vi "acc_gyro_motor_logger.vi"() -> ()   [LabVIEW 2012]
uses:
  <vilib>/Instr/_visa.llb/VISA Configure Serial Port (Instr).vi
  acc_gyro_data.ctl
panel:
  out "return count":u32
  in  "stop 2":bool
  out "Encoder":u8[](graph)
  in  "amp":dbl
  in  "freq":dbl
  in  "Send":bool
  in  "encoder counts per rev":dbl=2048.0
  in  "Motor serial port":refnum<visa-resource-name>="COM3"
  out "Rate":dbl[unit]
  out "Accelerometer":waveform(dbl)[](graph)
  out "Gyro":waveform(dbl)[](graph)
  in  "accel range (m/s2)":dbl(ring)=8.0 items=["2"=2.0, "4"=4.0, "8"=8.0, "16"=16.0]
  in  "gyro range (deg/s)":dbl(ring)=250.0 items=["250"=250.0, "500"=500.0, "1000"=1000.0, "2000"=2000.0]
  in  "Accelometer serial port":refnum<visa-resource-name>="COM3"
  in  "stop":bool
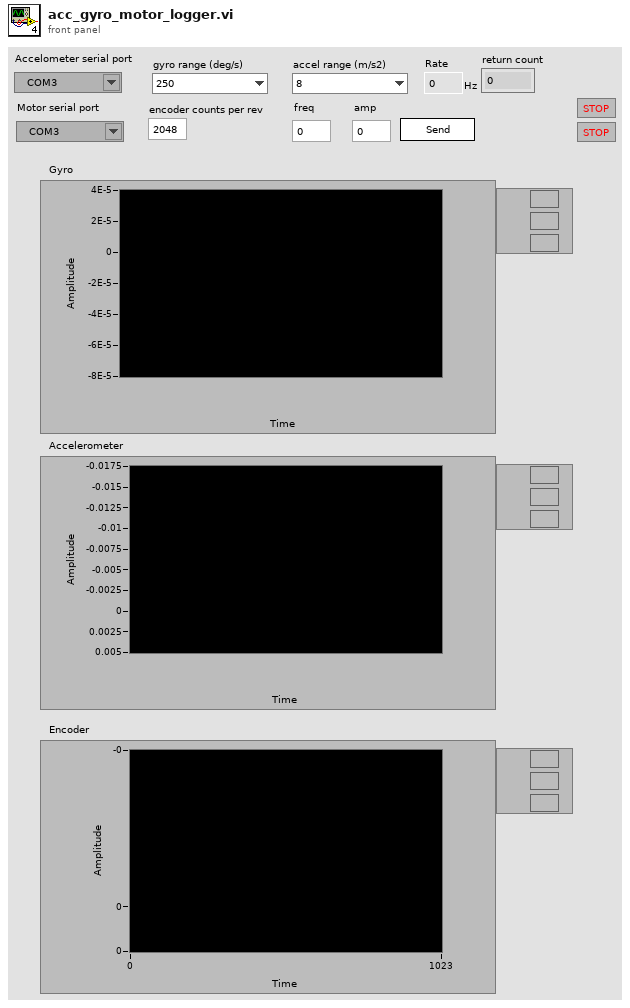
[diagram p1: front panel]
types:
  T1 = typedef "acc_gyro_data.ctl" = cluster{"milliseconds":u64, "gyro_x":dbl, "gyro_y":dbl, "gyro_z":dbl, "acc_x":dbl, "acc_y":dbl, "acc_z":dbl}
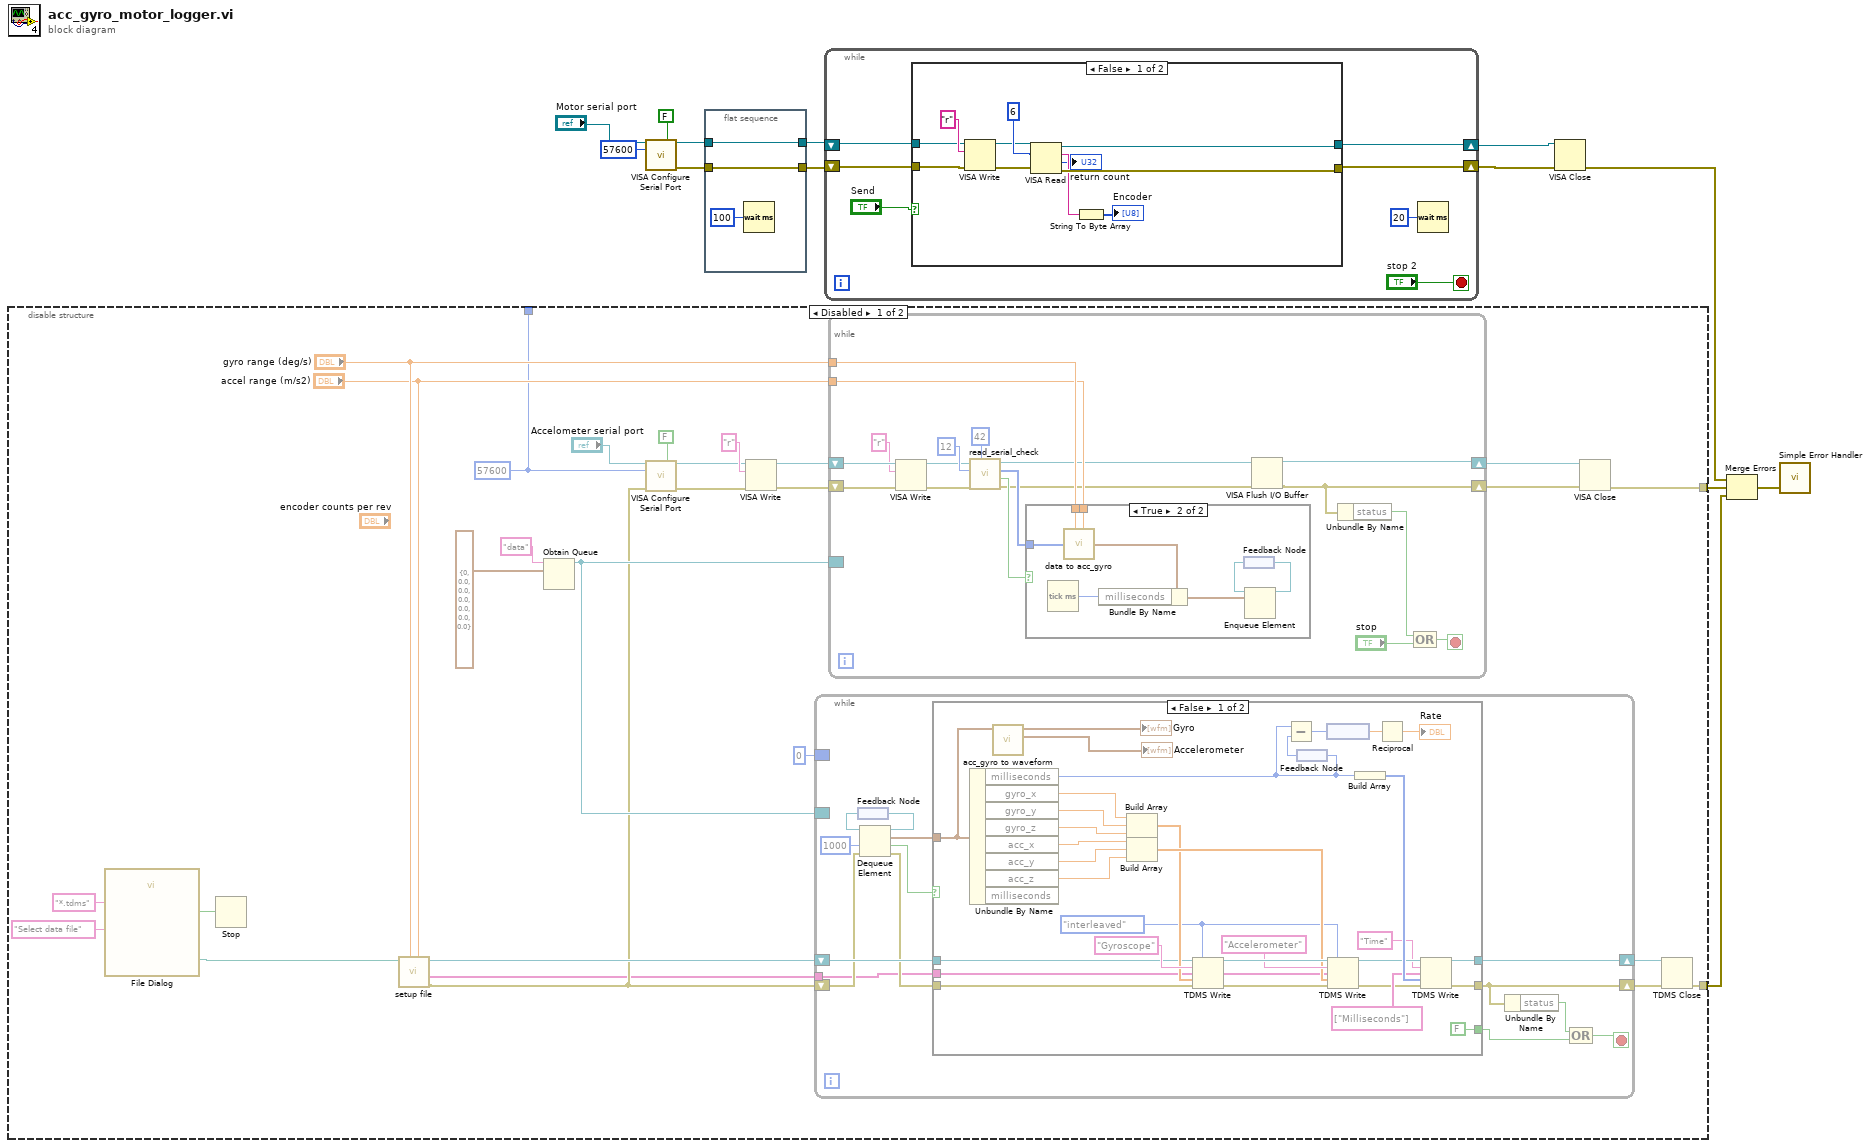
[diagram p0: block diagram]
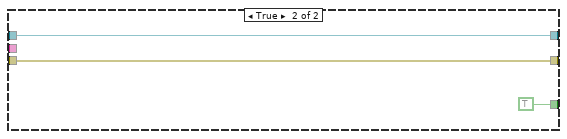
[diagram p2: hidden frame]
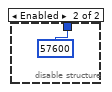
[diagram p4: hidden frame]
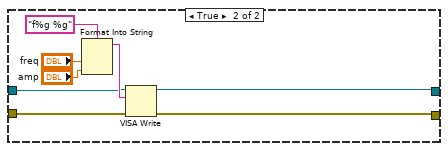
[diagram p5: hidden frame]
diagram:
  n1 = disable-structure shown="Disabled" {
    disable-tunnel: [w27 _] -> w13
    disable-tunnel: [w26 _] -> w12
    disable-tunnel: [w14 u32 57600 ("Baud rate")] -> _
    frame Disabled {
      w14 = u32 57600 ("Baud rate")
      n2 = call "File Dialog"("prompt"="Select data file", "pattern (all files)"="*.tdms") -> ("selected path"=w34:path, "cancelled"=w33:bool)  [unwired: 10 in, 2 out]
      n3 = Stop(stop? (T)=w33) -> ()
      n4 = call "setup file.vi"("accel range"="accel range (m/s2)", "gyro range"="gyro range (deg/s)", "selected path"=w34) -> ("error out"=w24:errorcluster, "channel names"=w21:string[], "tdms file out"=w25:refnum<k34>)  [unwired: 6 in]
      n5 = Obtain Queue(name (unnamed)="data", element data type=T1 {"milliseconds"=0, "gyro_x"=0.0, "gyro_y"=0.0, "gyro_z"=0.0, "acc_x"=0.0, "acc_y"=0.0, "acc_z"=0.0} ("acc gyro data")) -> (queue out=w32:refnum<queue>)  [unwired: 3 in, 2 out]
      n6 = call-poly "VISA Configure Serial Port"("VISA resource name"="Accelometer serial port", "Enable Termination\nChar (T)"=FALSE ("Enable Termination\nChar (T)"), "baud rate (9600)"=w14, "error in (no error)"=w24) -> ("VISA resource name out"=w18:refnum<visa-resource-name>, "error out"=w17:errorcluster)  [unwired: 10 in]
      n7 = VISA Write(VISA resource name=w18, write buffer="r", error in (no error)=w17) -> (VISA resource name out=w16:refnum<visa-resource-name>, error out=w15:errorcluster)  [unwired: 1 out]
      n8 = while {
        border: w32 -> [_]
        shift-right: [w45] -> w29
        shift-left: w24 -> [w48]
        shift-right: [w50] -> w28
        shift-left: w25 -> [w51]
        tunnel: w21 -> [w41]
        border: u64 0 ("milliseconds") -> [_]
        stop <- w42 stop-if-true
        n9 = feedback #1() -> (w54:refnum<queue>)
        n10 = Dequeue Element(queue=w54, timeout in ms (-1)=1000, error in (no error)=w48) -> (queue out=w53:refnum<queue>, element=w52:T1, timed out?=w46:bool, error out=w47:errorcluster)
        n11 = feedback-in #1(w53) -> ()
        n12 = case shown="False" w46 {
          tunnel: w52 -> [w72 _]
          tunnel: [w63 w88] -> w45
          tunnel: w51 -> [w61 w89]
          tunnel: [w62 w89] -> w50
          tunnel: w47 -> [w64 w88]
          tunnel: [FALSE TRUE] -> w43
          tunnel: w41 -> [w69 _]
          frame False {
            w60 = enum16{"decimated", "interleaved"}."interleaved" ("data layout (0:decimated)")
            n13 = Unbundle By Name(w72) -> ("milliseconds"=w59:u64, "gyro_x"=w87:dbl, "gyro_y"=w86:dbl, "gyro_z"=w85:dbl, "acc_x"=w84:dbl, "acc_y"=w83:dbl, "acc_z"=w82:dbl)  [unwired: 1 out]
            n14 = call "acc_gyro to waveform.vi"("acc gyro data"=w72) -> ("accel plot"=→"Accelerometer":waveform(dbl)[], "gyro plot"=→"Gyro":waveform(dbl)[])  [unwired: 9 in]
            n15 = Build Array(w87, w86, w85) -> (w73:dbl[])
            n16 = Build Array(w84, w83, w82) -> (w77:dbl[])
            n17 = TDMS Write(0:w61, 1:w60, 5:"Gyroscope" ("group name (Untitled)"), 7:w69, 9:w73, 11:w64) -> (4:w80:refnum<k34>, 8:w68:string[], 15:w79:errorcluster)  [unwired: 1 out]
            n18 = feedback #2() -> (w58:u64)
            n19 = Subtract(x=w59, y=w58) -> (x-y=w57:u64)
            n20 = feedback-in #2(w59) -> ()
            n21 = node(w57) -> (w56:dbl[unit])
            n22 = TDMS Write(0:w80, 1:w60, 5:"Accelerometer" ("group name (Untitled)"), 7:w68, 9:w77, 11:w79) -> (4:w67:refnum<k34>, 15:w66:errorcluster)  [unwired: 2 out]
            n23 = Build Array(w59) -> (w76:u64[])
            n24 = Reciprocal(x=w56) -> (1/x=→"Rate":dbl[unit])
            n25 = TDMS Write(0:w67, 5:"Time" ("group name (Untitled)"), 7:string[] ["Milliseconds"] ("channel name(s) in (Untitled)"), 9:w76, 11:w66) -> (4:w62:refnum<k34>, 15:w63:errorcluster)  [unwired: 1 in, 2 out]
          }
          frame True {
          }
        }
        n26 = Unbundle By Name(w45) -> ("status"=w44:bool)
        n27 = Compound Arithmetic op=OR(w44, w43) -> (w42:bool)
      }
      n28 = while {
        tunnel: "gyro range (deg/s)" -> [w103]
        tunnel: "accel range (m/s2)" -> [w102]
        border: w32 -> [_]
        shift-right: [w91] -> w31
        shift-left: w15 -> [w99]
        shift-right: [w93] -> w30
        shift-left: w16 -> [w108]
        stop <- w96 stop-if-true
        n29 = VISA Write(VISA resource name=w108, write buffer="r", error in (no error)=w99) -> (VISA resource name out=w101:refnum<visa-resource-name>, error out=w98:errorcluster)  [unwired: 1 out]
        n30 = call "read_serial_check.vi"("checkval"=u8 42, "error in (no error)"=w98, "byte count"=u32 12, "VISA resource name"=w101) -> ("error out"=w92:errorcluster, "good"=w105:bool, "data"=w104:u8[], "VISA resource out"=w94:refnum<visa-resource-name>)  [unwired: 4 in]
        n31 = case shown="True" w105 {
          tunnel: w104 -> [_ w116]
          tunnel: w103 -> [_ w115]
          tunnel: w102 -> [_ w114]
          frame False {
          }
          frame True {
            n32 = Tick Count (ms)() -> (millisecond timer value=w111:u32)
            n33 = call "data to acc_gyro.vi"("byte array"=w116, "gyro range (deg/s)"=w115, "accel range (m/s2)"=w114) -> ("acc gyro data"=w110:T1)
            n34 = Bundle By Name(cluster=w110, "milliseconds"=w111) -> (w109:T1)
            n35 = feedback #3() -> (w112:refnum<queue>)
            n36 = Enqueue Element(queue=w112, element=w109) -> (queue out=w113:refnum<queue>)  [unwired: 2 in, 2 out]
            n37 = feedback-in #3(w113) -> ()
          }
        }
        n38 = VISA Flush I/O Buffer(VISA resource name=w94, error in (no error)=w92) -> (VISA resource name out=w93:refnum<visa-resource-name>, error out=w91:errorcluster)  [unwired: 1 in]
        n39 = Unbundle By Name(w91) -> ("status"=w95:bool)
        n40 = Compound Arithmetic op=OR(w95, "stop") -> (w96:bool)
      }
      n41 = VISA Close(VISA resource name=w30, error in (no error)=w31) -> (error out=w27:errorcluster)
      n42 = TDMS Close(8:w29, 11:w28) -> (0:w26:errorcluster)  [unwired: 1 out]
    }
    frame Enabled {
    }
  }
  n43 = call-poly "VISA Configure Serial Port"("VISA resource name"="Motor serial port", "Enable Termination\nChar (T)"=FALSE ("Enable Termination\nChar (T)"), "baud rate (9600)"=u32 57600) -> ("VISA resource name out"=w5:refnum<visa-resource-name>, "error out"=w3:errorcluster)  [unwired: 11 in]
  n44 = flat-sequence {
    tunnel: w5 -> [w119]
    tunnel: [w119] -> w4
    tunnel: w3 -> [w118]
    tunnel: [w118] -> w2
    frame #0 {
      n45 = Wait (ms)(milliseconds to wait=u32 100) -> ()  [unwired: 1 out]
    }
  }
  n46 = while {
    shift-right: [w123] -> w7
    shift-left: w2 -> [w125]
    shift-right: [w124] -> w8
    shift-left: w4 -> [w126]
    stop <- "stop 2" stop-if-true
    n47 = case shown="False" "Send" {
      tunnel: w126 -> [w137 w142]
      tunnel: w125 -> [w136 w141]
      tunnel: [w132 w140] -> w124
      tunnel: [w131 w139] -> w123
      frame False {
        n48 = VISA Write(VISA resource name=w137, write buffer="r", error in (no error)=w136) -> (VISA resource name out=w134:refnum<visa-resource-name>, error out=w133:errorcluster)  [unwired: 1 out]
        n49 = VISA Read(VISA resource name=w134, byte count=u32 6, error in (no error)=w133) -> (VISA resource name out=w132:refnum<visa-resource-name>, read buffer=w130:string, return count=→"return count":u32, error out=w131:errorcluster)
        n50 = String To Byte Array(string=w130) -> (unsigned byte array=→"Encoder":u8[])
      }
      frame True {
        n51 = Format Into String(format string="f%g %g", "freq", "amp") -> (resulting string=w143:string)  [unwired: 2 in, 1 out]
        n52 = VISA Write(VISA resource name=w142, write buffer=w143, error in (no error)=w141) -> (VISA resource name out=w140:refnum<visa-resource-name>, error out=w139:errorcluster)  [unwired: 1 out]
      }
    }
    n53 = Wait (ms)(milliseconds to wait=u32 20) -> ()  [unwired: 1 out]
  }
  n54 = VISA Close(VISA resource name=w8, error in (no error)=w7) -> (error out=w6:errorcluster)
  n55 = Merge Errors(w6, w13, w12) -> (w11:errorcluster)
  n56 = call <vilib>:"Simple Error Handler.vi"("error in (no error)"=w11) -> ()  [unwired: 4 in, 5 out]
